vi "2d array to file.vi"(7 "file path (dialog if empty)":path, 8 "error in (no error)":errorcluster, 11 "Input":dbl[][](array[numeric])) -> (0 "error out":errorcluster)   [LabVIEW 2023]
uses:
  <vilib>/Utility/file.llb/Write Delimited Spreadsheet (DBL).vi
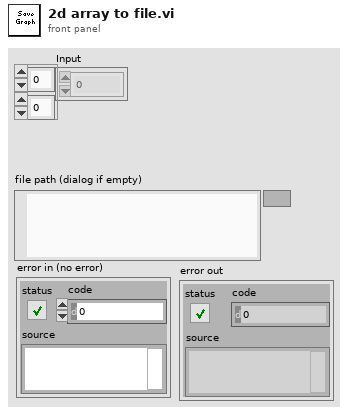
[diagram p1: front panel]
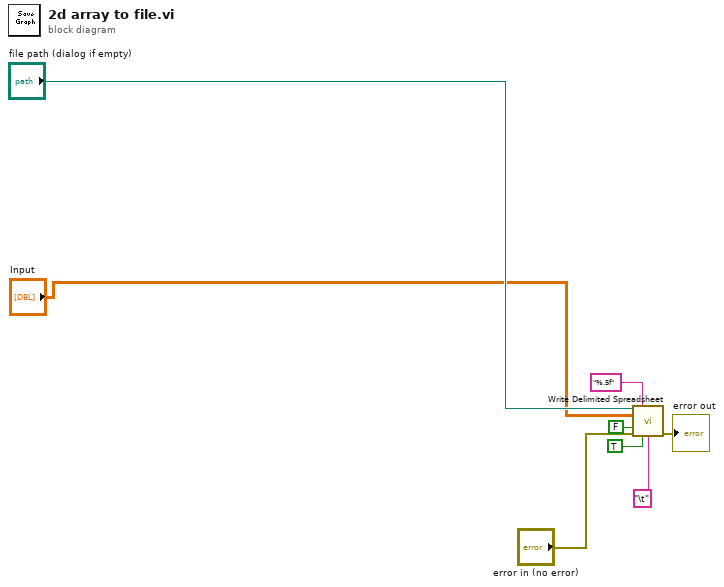
[diagram p0: block diagram]
diagram:
  n1 = call-poly <vilib>:"Write Delimited Spreadsheet.vi"("file path (dialog if empty)"="file path (dialog if empty)", "format (%.3f)"="%.5f", "2D data"="Input", "append to file? (new file:F)"=FALSE, "error in (no error)"="error in (no error)", "transpose? (no:F)"=TRUE, "delimiter (\\t)"="\t" ("delimiter (\\t)")) -> ("error out"=→"error out":errorcluster)  [unwired: 7 in, 1 out]
